vi "Override To Nominal State.vi"(11 "Base Event in":refnum<class "Base Event.lvclass">) -> (3 "Base Event out":refnum<class "Base Event.lvclass">)   [LabVIEW 2021, in "jettl.lvlib" / "Base Event.lvlib" / "Base Event.lvclass"]
uses:
  Base Event.lvclass
  State/Nominal State/Nominal State.lvclass
  C:/git/jettl/jettl/jettl/Base Event/State/State/State.lvclass
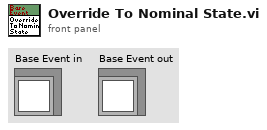
[diagram p1: front panel]
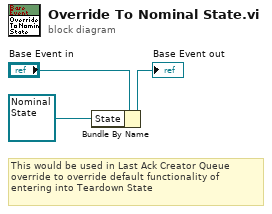
[diagram p0: block diagram]
diagram:
  # "This would be used in Last Ack Creator Queue override to override default functionality of entering into Teardown State"
  n1 = Bundle By Name(cluster="Base Event in", "State"=refnum<class "Nominal State.lvclass"> refnum ("jettl.lvlib:Base Event.lvlib:State.lvlib:Nominal State.lvclass")) -> (→"Base Event out":refnum<class "Base Event.lvclass">)
